vi "Lab Panel V5.10.vi"() -> ()   [LabVIEW 2013]
uses:
  <vilib>/Platform/TimedLoop/XDataNode/timing_clust.ctl
  <vilib>/Platform/TimedLoop/XDataNode/nitl_modes.ctl
  <vilib>/Platform/TimedLoop/XDataNode/wakeup.ctl
  Global display 4.vi
  Global display 3.vi
  Global display 1.vi
  Global 1.vi
  Global display 2.vi
  <vilib>/platform/TimedLoop/XDataNode/XDataNode.xnode
  <vilib>/Platform/TimedLoop/XDataNode/XDNodeRunTimeDep.lvlib
panel:
  out "Simulate IND":bool
  out "Amb Tp":dbl format="%#.0f"
  out "Tp Ut":dbl
  out "network error":bool
  out "TEMP":bool
  out "AI":bool
  in  "stop all":bool
  in  "ADMIN":bool
  in  "Tab Control 2":T1(tab)
  out "SIG LAB05-2":T2 {"PF" format="%.2f"; "AMPS" format="%.1f"}
  out "SIG LAB05-1":T2 {"PF" format="%.2f"; "AMPS" format="%.1f"}
  out "SIG LAB04-2":T2 {"PF" format="%.2f"; "AMPS" format="%.1f"}
  out "SIG LAB04-1":T2 {"PF" format="%.2f"; "AMPS" format="%.1f"}
  out "SIG LAB03-2":T2 {"PF" format="%.2f"; "AMPS" format="%.1f"}
  out "SIG LAB03-1":T2 {"PF" format="%.2f"; "AMPS" format="%.1f"}
  out "SIG LAB02-2":T2 {"PF" format="%.2f"; "AMPS" format="%.1f"}
  in  "RUN LAB01-1":bool
  in  "O/I  LAB05-1":bool
  in  "O/I  LAB05-2":bool
  in  "O/I  LAB04-1":bool
  in  "O/I  LAB04-2":bool
  in  "O/I  LAB02-1":bool
  in  "O/I  LAB02-2":bool
  in  "O/I  LAB01-2":bool
  in  "O/I  LAB01-1":bool
  in  "O/I  LAB03-1":bool
  in  "RUN LAB05-2":bool
  in  "RUN LAB05-1":bool
  in  "RUN LAB04-2":bool
  in  "RUN LAB04-1":bool
  in  "RUN LAB03-2":bool
  in  "RUN LAB03-1":bool
  in  "RUN LAB02-2":bool
  in  "RUN LAB02-1":bool
  in  "RUN LAB01-2":bool
  in  "SELECT LAB05-2":T3(radio)
  in  "SELECT LAB05-1":T3(radio)
  in  "SELECT LAB04-2":T3(radio)
  in  "SELECT LAB04-1":T3(radio)
  in  "SELECT LAB03-2":T3(radio)
  in  "SELECT LAB03-1":T3(radio)
  in  "SELECT LAB02-2":T3(radio)
  in  "SELECT LAB02-1":T3(radio)
  in  "SELECT LAB01-2":T3(radio)
  in  "SELECT LAB01-1":T3(radio)
  in  "O/I  LAB03-2":bool
  out "SIG LAB01-1":T2 {"PF" format="%.2f"; "AMPS" format="%.1f"}
  out "SIG LAB01-2":T2 {"PF" format="%.2f"; "AMPS" format="%.1f"}
  out "SIG LAB02-1":T2 {"PF" format="%.2f"; "AMPS" format="%.1f"}
  out "DISP LAB05-2":T4 {"MINS" format="%.2g"}
  out "DISP LAB05-1":T4 {"MINS" format="%.2g"}
  out "DISP LAB04-2":T4 {"MINS" format="%.2g"}
  out "DISP LAB04-1":T4 {"MINS" format="%.2g"}
  out "DISP LAB03-2":T4 {"MINS" format="%.2g"}
  out "DISP LAB03-1":T4 {"MINS" format="%.2g"}
  in  "SET LAB05-2":T5={"NAME"="", "DESCRIPTION"="", "CYCLES"=5.0, "T-RISE mins"=0.0, "T-RISE deg C"=0.0} {"CYCLES" min=5.0 step=1.0}
  in  "SET LAB05-1":T5={"NAME"="", "DESCRIPTION"="", "CYCLES"=5.0, "T-RISE mins"=0.0, "T-RISE deg C"=0.0} {"CYCLES" min=5.0 step=1.0}
  in  "SET LAB04-2":T5={"NAME"="", "DESCRIPTION"="", "CYCLES"=5.0, "T-RISE mins"=0.0, "T-RISE deg C"=0.0} {"CYCLES" min=5.0 step=1.0}
  in  "SET LAB04-1":T5={"NAME"="", "DESCRIPTION"="", "CYCLES"=5.0, "T-RISE mins"=0.0, "T-RISE deg C"=0.0} {"CYCLES" min=5.0 step=1.0}
  in  "SET LAB03-2":T5={"NAME"="", "DESCRIPTION"="", "CYCLES"=5.0, "T-RISE mins"=0.0, "T-RISE deg C"=0.0} {"CYCLES" min=5.0 step=1.0}
  in  "SET LAB03-1":T5={"NAME"="", "DESCRIPTION"="", "CYCLES"=5.0, "T-RISE mins"=0.0, "T-RISE deg C"=0.0} {"CYCLES" min=5.0 step=1.0}
  out "DISP LAB02-2":T4 {"MINS" format="%.2g"}
  out "DISP LAB02-1":T4 {"MINS" format="%.2g"}
  in  "SET LAB02-2":T5={"NAME"="", "DESCRIPTION"="", "CYCLES"=5.0, "T-RISE mins"=0.0, "T-RISE deg C"=0.0} {"CYCLES" min=5.0 step=1.0}
  in  "SET LAB02-1":T5={"NAME"="", "DESCRIPTION"="", "CYCLES"=5.0, "T-RISE mins"=0.0, "T-RISE deg C"=0.0} {"CYCLES" min=5.0 step=1.0}
  out "RESULT LAB05-2":bool
  out "RESULT LAB05-1":bool
  out "RESULT LAB04-2":bool
  out "RESULT LAB04-1":bool
  out "RESULT LAB03-2":bool
  out "RESULT LAB03-1":bool
  out "RESULT LAB02-2":bool
  out "RESULT LAB02-1":bool
  out "RESULT LAB01-2":bool
  out "RESULT LAB01-1":bool
  in  "SET LAB01-1":T5={"NAME"="", "DESCRIPTION"="", "CYCLES"=5.0, "T-RISE mins"=0.0, "T-RISE deg C"=0.0} {"CYCLES" min=5.0 step=1.0}
  in  "SET LAB01-2":T5={"NAME"="", "DESCRIPTION"="", "CYCLES"=5.0, "T-RISE mins"=0.0, "T-RISE deg C"=0.0} {"CYCLES" min=5.0 step=1.0}
  out "DISP LAB01-1":T4 {"MINS" format="%.2g"}
  out "DISP LAB01-2":T4 {"MINS" format="%.2f"}
  out "TEMP RISE LAB05-2":cluster{"TL":dbl, "TN":dbl}
  out "TEMP RISE LAB05-1":cluster{"TL":dbl, "TN":dbl}
  out "TEMP RISE LAB04-2":cluster{"TL":dbl, "TN":dbl}
  out "TEMP RISE LAB04-1":cluster{"TL":dbl, "TN":dbl}
  out "TEMP RISE LAB03-2":cluster{"TL":dbl, "TN":dbl}
  out "TEMP RISE LAB03-1":cluster{"TL":dbl, "TN":dbl}
  out "TEMP RISE LAB02-2":cluster{"TL":dbl, "TN":dbl}
  out "TEMP RISE LAB02-1":cluster{"TL":dbl, "TN":dbl}
  out "TEMP RISE LAB01-2":cluster{"TL":dbl, "TN":dbl}
  out "TEMP RISE LAB01-1":cluster{"TL":dbl, "TN":dbl}
  out "JIG LAB05-2":bool
  out "JIG LAB05-1":bool
  out "JIG LAB04-2":bool
  out "JIG LAB04-1":bool
  out "JIG LAB03-2":bool
  out "JIG LAB03-1":bool
  out "JIG LAB02-2":bool
  out "JIG LAB02-1":bool
  out "JIG LAB01-2":bool
  out "JIG LAB01-1":bool
  out "TEMP START LAB01-1":cluster{"TL":dbl, "TN":dbl}
  out "TEMP START LAB02-1":cluster{"TL":dbl, "TN":dbl}
  out "TEMP START LAB03-1":cluster{"TL":dbl, "TN":dbl}
  out "TEMP START LAB04-1":cluster{"TL":dbl, "TN":dbl}
  out "TEMP START LAB01-2":cluster{"TL":dbl, "TN":dbl}
  out "TEMP START LAB02-2":cluster{"TL":dbl, "TN":dbl}
  out "TEMP START LAB03-2":cluster{"TL":dbl, "TN":dbl}
  out "TEMP START LAB04-2":cluster{"TL":dbl, "TN":dbl}
  out "TEMP START LAB05-2":cluster{"TL":dbl, "TN":dbl}
  out "TEMP START LAB05-1":cluster{"TL":dbl, "TN":dbl}
  out "LOG LAB05-2":string
  out "LOG LAB04-2":string
  out "LOG LAB03-2":string
  out "LOG LAB02-2":string
  out "LOG LAB01-2":string
  out "LOG LAB05-1":string
  out "LOG LAB04-1":string
  out "LOG LAB03-1":string
  out "LOG LAB02-1":string
  out "LOG LAB01-1":string
  in  "Tab charts":T6(tab)
  out "LAB01 VOLTS":dynamicdata(graph)
  out "LAB01 AMPS":dynamicdata(graph)
  out "LAB01 deg C":dynamicdata(graph)
  out "LAB02 VOLTS":dynamicdata(graph)
  out "LAB02 AMPS":dynamicdata(graph)
  out "LAB02 deg C":dynamicdata(graph)
  out "LAB03 VOLTS":dynamicdata(graph)
  out "LAB03 AMPS":dynamicdata(graph)
  out "LAB03 deg C":dynamicdata(graph)
  out "LAB04 VOLTS":dynamicdata(graph)
  out "LAB04 AMPS":dynamicdata(graph)
  out "LAB04 deg C":dynamicdata(graph)
  out "LAB05 VOLTS":dynamicdata(graph)
  out "LAB05 AMPS":dynamicdata(graph)
  out "LAB05 deg C":dynamicdata(graph)
  out "Resets Done":dbl
  out "Error USB #2":bool
  out "Error USB #1":bool
  out "Error USB #0":bool
  in  "MAIL SETTINGS":T7
  out "MAIL REPORT":string
  in  "TO (string):":string
  in  "Send Mail Now":bool
  in  "Auto Mail Send":bool
  in  "Network Directory":path
  in  "JIG ON TIME (S)":dbl=1.0 min=1.0 max=10.0 step=0.5 format="%.1g"
  in  "JIG OFF TIME (S)":dbl=2.0 min=2.0 max=10.0 step=0.5 format="%.1g"
  in  "Reset Measuring":bool
  out "JIG RELAY CYCLES":T8
  out "ON L05-2":cluster{"amps":dbl, "volts":dbl, "pf":dbl}
  out "ON L05-1":cluster{"amps":dbl, "volts":dbl, "pf":dbl}
  out "FAIL LAB05-2":cluster{"LO":dbl, "HI":dbl}
  out "FAIL LAB05-1":cluster{"LO":dbl, "HI":dbl}
  out "FAIL LAB04-2":cluster{"LO":dbl, "HI":dbl}
  out "FAIL LAB04-1":cluster{"LO":dbl, "HI":dbl}
  out "FAIL LAB03-2":cluster{"LO":dbl, "HI":dbl}
  out "FAIL LAB03-1":cluster{"LO":dbl, "HI":dbl}
  out "FAIL LAB02-2":cluster{"LO":dbl, "HI":dbl}
  out "FAIL LAB02-1":cluster{"LO":dbl, "HI":dbl}
  out "FAIL LAB01-2":cluster{"LO":dbl, "HI":dbl}
  out "FAIL LAB01-1":cluster{"LO":dbl, "HI":dbl}
  out "ON L01-1":cluster{"amps":dbl, "volts":dbl, "pf":dbl}
  out "ON L01-2":cluster{"amps":dbl, "volts":dbl, "pf":dbl}
  out "ON L02-1":cluster{"amps":dbl, "volts":dbl, "pf":dbl}
  out "ON L02-2":cluster{"amps":dbl, "volts":dbl, "pf":dbl}
  out "ON L03-1":cluster{"amps":dbl, "volts":dbl, "pf":dbl}
  out "ON L03-2":cluster{"amps":dbl, "volts":dbl, "pf":dbl}
  out "ON L04-1":cluster{"amps":dbl, "volts":dbl, "pf":dbl}
  out "ON L04-2":cluster{"amps":dbl, "volts":dbl, "pf":dbl}
  out "TEMP LA05":T9
  out "TEMP LA04":T9
  out "TEMP LA03":T9
  out "TEMP LA02":T9
  out "TEMP LA01":T9
  out "Ref deg C":dbl format="%#.0f"
  out "Panel #":dbl
  in  "Mail Test File To:":string
  in  "Mail Test Fail":bool
  out "graph flag":bool
  in  "Temp Test Cal":dbl
  in  "Amps Fail level":dbl
  in  "Fail Loops":dbl
  out "Save JC":bool
  out "simulate":bool
  in  "Temp Value":dbl
  in  "Temp Delay Lps":dbl
  in  "SAMPLES":dbl
  in  "RATE (Hz)":dbl
  in  "JIG TEST":T10
  in  "C drive data root dir":path
  out "run lab05-2":bool
  out "run lab05-1":bool
  out "run lab04-2":bool
  out "run lab04-1":bool
  out "run lab03-2":bool
  out "run lab03-1":bool
  out "run lab02-2":bool
  out "run lab02-1":bool
  out "run lab01-2":bool
  out "run lab01-1":bool
  in  "Tab Control":T11(tab)
  out "LAB01-2 (GRAPH)":dynamicdata(graph)
  out "LAB01-1 (GRAPH)":dynamicdata(graph)
  out "LAB02-2 (GRAPH)":dynamicdata(graph)
  out "LAB02-1 (GRAPH)":dynamicdata(graph)
  out "LAB03-2 (GRAPH)":dynamicdata(graph)
  out "LAB03-1 (GRAPH)":dynamicdata(graph)
  out "LAB04-2 (GRAPH)":dynamicdata(graph)
  out "LAB04-1 (GRAPH)":dynamicdata(graph)
  out "LAB05-2 (GRAPH)":dynamicdata(graph)
  out "LAB05-1 (GRAPH)":dynamicdata(graph)
  out "LAB05 TEMP":T12
  out "LAB04 TEMP":T12
  out "LAB02 TEMP":T12
  out "LAB01 TEMP":T12
  out "LAB03 TEMP":T12
  out "Analog error":bool
  in  "Ambient Volts":dbl format="%.2f"
  in  "PF":dbl min=0.0 max=1.0 step=0.1 format="%#.1f"
  in  "VOLTS":dbl
  in  "OFF amps":dbl min=0.0 max=100.0 step=0.1 format="%#.1f"
  in  "ON amps":dbl
  in  "LAB deg C":T13
  out "AI loop time":dbl format="%.6g"
  out "loops":dbl
  in  "loop  delay(mS)":dbl
  out "on loops":dbl
  out "off loops":dbl
  out "jig cycle":dbl
  out "TDMS LAB01-1":refnum<k34>
  out "data file error":errorcluster
  out "TDMS LAB02-1":refnum<k34>
  out "TDMS LAB01-2":refnum<k34>
  out "TDMS LAB02-2":refnum<k34>
  out "TDMS LAB03-1":refnum<k34>
  out "TDMS LAB03-2":refnum<k34>
  out "TDMS LAB04-1":refnum<k34>
  out "TDMS LAB04-2":refnum<k34>
  out "TDMS LAB05-1":refnum<k34>
  out "TDMS LAB05-2":refnum<k34>
  out "mail control":string
  out "File Time Stamp":timestamp
  in  "stop":bool
  in  "Select COM port":refnum<visa-resource-name>="COM6"
  out "COM port":refnum<visa-resource-name>="COM6"
  out "deg C (volts)":dbl
  out "TEMP REF cal":dbl
  out "CAL LAB01":T14 {"2 (TN) cal" min=0.0 step=0.01 format="%.2f"; "2 (TL) cal" min=0.0 step=0.01 format="%.2f"; "2 (PF) cal" min=0.0 step=0.01 format="%.2f"; "2 (V) cal" min=0.0 step=0.01 format="%.2f"; "2 (A) cal" min=0.0 step=0.01 format="%.2f"; "1 (TN) cal" min=0.0 step=0.01 format="%.2f"; "1 (TL) cal" min=0.0 step=0.01 format="%.2f"; "1 (PF) cal" min=0.0 step=0.01 format="%.2f"; "1 (V) cal" min=0.0 step=0.01 format="%.2f"; "1  (A) cal" min=0.0 step=0.01 format="%.2f"}
  out "CAL LAB03":T14 {"2 (TN) cal" min=0.0 step=0.01 format="%.2f"; "2 (TL) cal" min=0.0 step=0.01 format="%.2f"; "2 (PF) cal" min=0.0 step=0.01 format="%.2f"; "2 (V) cal" min=0.0 step=0.01 format="%.2f"; "2 (A) cal" min=0.0 step=0.01 format="%.2f"; "1 (TN) cal" min=0.0 step=0.01 format="%.2f"; "1 (TL) cal" min=0.0 step=0.01 format="%.2f"; "1 (PF) cal" min=0.0 step=0.01 format="%.2f"; "1 (V) cal" min=0.0 step=0.01 format="%.2f"; "1  (A) cal" min=0.0 step=0.01 format="%.2f"}
  out "CAL LAB02":T15 {"2 (TN) cal" min=0.0 step=0.01 format="%.2f"; "2 (TL) cal" min=0.0 step=0.01 format="%.2f"; "2 (PF) cal" min=0.0 step=0.01 format="%.2f"; "2 (V) cal" min=0.0 step=0.01 format="%.2f"; "2 (A) cal" min=0.0 step=0.01 format="%.2f"; "1 (TN) cal" min=0.0 step=0.01 format="%.2f"; "1 (TL) cal" min=0.0 step=0.01 format="%.2f"; "1 (PF) cal" min=0.0 step=0.01 format="%.2f"; "1 (V) cal" min=0.0 step=0.01 format="%.2f"; "1 (A) cal" min=0.0 step=0.01 format="%.2f"}
  out "CAL LAB05":T14 {"2 (TN) cal" min=0.0 step=0.01 format="%.2f"; "2 (TL) cal" min=0.0 step=0.01 format="%.2f"; "2 (PF) cal" min=0.0 step=0.01 format="%.2f"; "2 (V) cal" min=0.0 step=0.01 format="%.2f"; "2 (A) cal" min=0.0 step=0.01 format="%.2f"; "1 (TN) cal" min=0.0 step=0.01 format="%.2f"; "1 (TL) cal" min=0.0 step=0.01 format="%.2f"; "1 (PF) cal" min=0.0 step=0.01 format="%.2f"; "1 (V) cal" min=0.0 step=0.01 format="%.2f"; "1  (A) cal" min=0.0 step=0.01 format="%.2f"}
  out "CAL LAB04":T14 {"2 (TN) cal" min=0.0 step=0.01 format="%.2f"; "2 (TL) cal" min=0.0 step=0.01 format="%.2f"; "2 (PF) cal" min=0.0 step=0.01 format="%.2f"; "2 (V) cal" min=0.0 step=0.01 format="%.2f"; "2 (A) cal" min=0.0 step=0.01 format="%.2f"; "1 (TN) cal" min=0.0 step=0.01 format="%.2f"; "1 (TL) cal" min=0.0 step=0.01 format="%.2f"; "1 (PF) cal" min=0.0 step=0.01 format="%.2f"; "1 (V) cal" min=0.0 step=0.01 format="%.2f"; "1  (A) cal" min=0.0 step=0.01 format="%.2f"}
  out "cal file error out":errorcluster
  in  "SET (cal)":bool
  # "LAB01"
  # "LAB02"
  # "LAB03"
  # "LAB04"
  # "LAB05"
  # "LAB01"
  # "LAB02"
  # "LAB03"
  # "LAB04"
  # "LAB05"
  # "PANEL ID / DATE / TIME / NAME / DESCRIPTION / CYCLES / TEST TIME / STATUS"
  # "PANEL ID / DATE / TIME / NAME / DESCRIPTION / CYCLES / TEST TIME / STATUS"
  # "(Enter recipients address seperated by comma)"
  # "JIG SET"
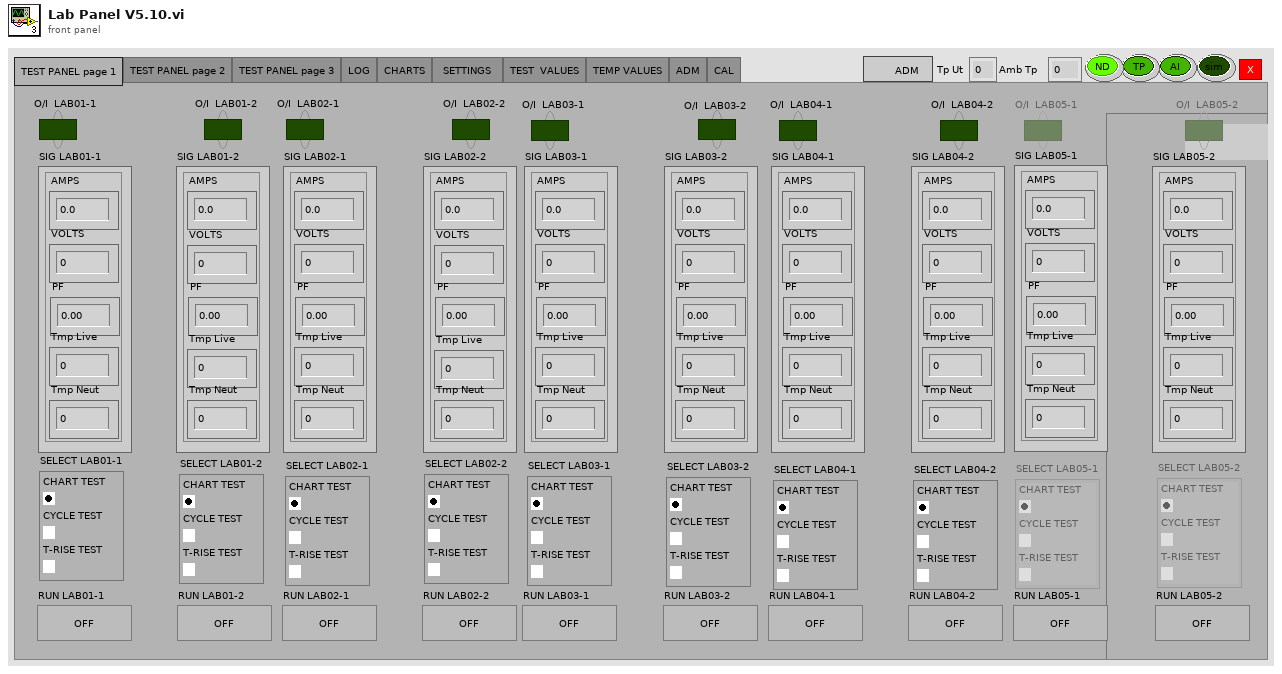
[diagram p1: front panel]
types:
  T1 = enum32{"TEST PANEL page 1", "TEST PANEL page 2", "TEST PANEL page 3", "LOG", "CHARTS", "SETTINGS   ", "TEST  VALUES", "TEMP VALUES", "ADM", "CAL"}
  T2 = cluster{"AMPS":dbl, "VOLTS":dbl, "PF":dbl, "Tmp Live":dbl, "Tmp Neut":dbl}
  T3 = enum32{"CHART TEST", "CYCLE TEST", "T-RISE TEST"}
  T4 = cluster{"CYCLE":dbl, "MINS":dbl, "STATUS":string}
  T5 = cluster{"NAME":string, "DESCRIPTION":string, "CYCLES":dbl, "T-RISE mins":dbl, "T-RISE deg C":dbl}
  T6 = enum32{"LAB01", "LAB02", "LAB03", "LAB04", "LAB05"}
  T7 = cluster{"OUT SERVER ADDRESS":string, "FROM ACCOUNT":string, "USER NAME":string, "PASSWORD":string, "TEST MAIL":bool, "TEST MAIL STATUS":string, "mail error":errorcluster}
  T8 = cluster{"LAB01-1":dbl, "LAB01-2":dbl, "LAB02-1":dbl, "LAB02-2":dbl, "LAB03-1":dbl, "LAB03-2":dbl, "LAB04-1":dbl, "LAB04-2":dbl, "LAB05-1":dbl, "LAB05-2":dbl}
  T9 = cluster{"TL-1":dbl, "TN-1":dbl, "TL-2":dbl, "TN-2":dbl, "TL -1COUNT":dbl, "TN-1 COUNT":dbl, "TL-2 COUNT":dbl, "TN-2 COUNT":dbl}
  T10 = cluster{" LAB01-1":bool, " LAB01-2":bool, "LAB02-1":bool, " LAB02-2":bool, "LAB03-1":bool, "LAB03-2":bool, "LAB04-1":bool, "LAB04-2":bool, "LAB05-1":bool, "LAB05-2":bool}
  T11 = enum32{"LAB01", "LAB02", "LAB03", "LAB04", "LAB05", "TEMPERATURE", "ERROR", "Simulate"}
  T12 = cluster{"T1 Live":dbl, "T1 Neut":dbl, "T2 Live":dbl, "T2 Neut":dbl, "ID":dbl, "ER":dbl}
  T13 = cluster{"1 TL":dbl, "1 TN":dbl, "2 TL":dbl, "2 TN":dbl, "ID":dbl, "ER":dbl}
  T14 = cluster{"1  (A) cal":dbl, "1 (V) cal":dbl, "1 (PF) cal":dbl, "1 (TL) cal":dbl, "1 (TN) cal":dbl, "2 (A) cal":dbl, "2 (V) cal":dbl, "2 (PF) cal":dbl, "2 (TL) cal":dbl, "2 (TN) cal":dbl}
  T15 = cluster{"1 (A) cal":dbl, "1 (V) cal":dbl, "1 (PF) cal":dbl, "1 (TL) cal":dbl, "1 (TN) cal":dbl, "2 (A) cal":dbl, "2 (V) cal":dbl, "2 (PF) cal":dbl, "2 (TL) cal":dbl, "2 (TN) cal":dbl}
  T16 = enum8{"Enabled", "Disabled", "Disabled and Grayed Out"}
  T17 = typedef "XDNodeRunTimeDep.lvlib/timing_clust.ctl" = cluster{"Expected End [f-1]":u64, "Actual End [f-1]":u64, "Finished Late? [f-1]":bool, "Expected End [i-1]":u64, "Actual End [i-1]":u64, "Finished Late? [i-1]":bool, "Expected Start [i]":u64, "Actual Start [i]":u64, "Expected Start [f]":u64, "Actual Start [f]":u64, "Source Name":string, "Structure Name":string, "Period":i64, "Deadline":i64, "Offset":i64, "Start":i64, "Priority":i32, "Timeout":i32, "Mode":T18, "Wakeup Reason":T19, "Error":errorcluster, "Source Type":string, "Secondary Source Type":string, "Global End Time":u64, "Global Start Time":u64, "Frame Duration":u64, "Iteration Duration":u64, "Assigned CPU":i32, "I/O Scan Engine Mode":u32}
  T18 = typedef "XDNodeRunTimeDep.lvlib/nitl_modes.ctl" = enum32{"No Change", "Process missed periods, maintain original phase", "Discard missed periods, maintain original phase", "Process missed periods, ignore original phase", "Discard missed periods, ignore original phase"}
  T19 = typedef "XDNodeRunTimeDep.lvlib/wakeup.ctl" = enum32{"Normal", "Aborted", "Asynchronous wakeup", "Timing source error", "Timed loop error", "Timeout"}
  T20 = enum16{"open", "open or create", "create or replace", "create", "open (read-only)"}
  T21 = enum16{"open", "replace", "create", "open or create", "replace or create", "replace or create with confirmation"}
  T22 = cluster{"SET LAB01-1":cluster{"NAME":string, "DESCRIPTION":string, "CYCLES":dbl, "T-RISE mins":dbl, "T-RISE deg C":dbl}, "SET LAB01-2":cluster{"NAME":string, "DESCRIPTION":string, "CYCLES":dbl, "T-RISE mins":dbl, "T-RISE deg C":dbl}, "SET LAB02-1":cluster{"NAME":string, "DESCRIPTION":string, "CYCLES":dbl, "T-RISE mins":dbl, "T-RISE deg C":dbl}, "SET LAB02-2":cluster{"NAME":string, "DESCRIPTION":string, "CYCLES":dbl, "T-RISE mins":dbl, "T-RISE deg C":dbl}, "SET LAB03-1":cluster{"NAME":string, "DESCRIPTION":string, "CYCLES":dbl, "T-RISE mins":dbl, "T-RISE deg C":dbl}, "SET LAB03-2":cluster{"NAME":string, "DESCRIPTION":string, "CYCLES":dbl, "T-RISE mins":dbl, "T-RISE deg C":dbl}, "SET LAB04-1":cluster{"NAME":string, "DESCRIPTION":string, "CYCLES":dbl, "T-RISE mins":dbl, "T-RISE deg C":dbl}, "SET LAB04-2":cluster{"NAME":string, "DESCRIPTION":string, "CYCLES":dbl, "T-RISE mins":dbl, "T-RISE deg C":dbl}, "SET LAB05-1":cluster{"NAME":string, "DESCRIPTION":string, "CYCLES":dbl, "T-RISE mins":dbl, "T-RISE deg C":dbl}, "SET LAB05-2":cluster{"NAME":string, "DESCRIPTION":string, "CYCLES":dbl, "T-RISE mins":dbl, "T-RISE deg C":dbl}, "Network Directory":path, "C drive data root dir":path, "RATE (Hz)":dbl, "SAMPLES":dbl, "Select COM port":refnum<visa-resource-name>, "Temp Delay Lps":dbl, "Temp Value":dbl, "Fail Loops":dbl, "Temp Test Cal":dbl, "Amps Fail level":dbl, "Mail Test File To:":string, "Mail Test Fail":bool}
  T23 = cluster{"MAIL SETTINGS":cluster{"OUT SERVER ADDRESS":string, "FROM ACCOUNT":string, "USER NAME":string, "PASSWORD":string, "TEST MAIL":bool, "TEST MAIL STATUS":string, "mail error":errorcluster}, "Auto Mail Send":bool, string}
  T24 = cluster{"T1":dbl, "T2":dbl, "T3":dbl, "T4":dbl, "ID":dbl, "ER":dbl}
  T25 = cluster{"STATUS":string, "OUT SERVER ADDRESS":string, "FROM ACCOUNT":string, "Mail Test File To:":string, "Mail Test Fail":bool}
  T26 = cluster{"LAB01-1 (A)":dbl, "LAB01-1 (V)":dbl, "LAB01-1 (PF)":dbl, "LAB01-2 (A)":dbl, "LAB01-2 (V)":dbl, "LAB01-2 (PF)":dbl}
  T27 = cluster{"LAB02-1 (A)":dbl, "LAB02-1 (V)":dbl, "LAB02-1 (PF)":dbl, "LAB02-2 (A)":dbl, "LAB02-2 (V)":dbl, "LAB02-2 (PF)":dbl}
  T28 = cluster{"LAB03-1 (A)":dbl, "LAB03-1 (V)":dbl, "LAB03-1 (PF)":dbl, "LAB03-2 (A)":dbl, "LAB03-2 (V)":dbl, "LAB03-2 (PF)":dbl}
  T29 = cluster{"LAB04-1 (A)":dbl, "LAB04-1 (V)":dbl, "LAB04-1 (PF)":dbl, "LAB04-2 (A)":dbl, "LAB04-2 (V)":dbl, "LAB04-2 (PF)":dbl}
  T30 = cluster{"LAB05-1 (A)":dbl, "LAB05-1 (V)":dbl, "LAB05-1 (PF)":dbl, "LAB05-2 (A)":dbl, "LAB05-2 (V)":dbl, "LAB05-2 (PF)":dbl}
  T31 = cluster{"OFF amps":dbl, "VOLTS":dbl, "PF":dbl, "OFF amps":dbl, "VOLTS":dbl, "PF":dbl}
  T32 = cluster{"FAIL LAB01-1":cluster{"LO":dbl, "HI":dbl}, "SIG LAB01-1":cluster{"AMPS":dbl, "VOLTS":dbl, "PF":dbl, "Tmp Live":dbl, "Tmp Neut":dbl}, "TEMP START LAB01-1":cluster{"TL":dbl, "TN":dbl}, "DISP LAB01-1":cluster{"CYCLE":dbl, "MINS":dbl, "STATUS":string}, "SET LAB01-1":cluster{"NAME":string, "DESCRIPTION":string, "CYCLES":dbl, "T-RISE mins":dbl, "T-RISE deg C":dbl}, "TDMS LAB01-1":refnum<k34>}
  T33 = cluster{"FAIL LAB01-2":cluster{"LO":dbl, "HI":dbl}, "SIG LAB01-2":cluster{"AMPS":dbl, "VOLTS":dbl, "PF":dbl, "Tmp Live":dbl, "Tmp Neut":dbl}, "TEMP START LAB01-2":cluster{"TL":dbl, "TN":dbl}, "DISP LAB01-2":cluster{"CYCLE":dbl, "MINS":dbl, "STATUS":string}, "SET LAB01-2":cluster{"NAME":string, "DESCRIPTION":string, "CYCLES":dbl, "T-RISE mins":dbl, "T-RISE deg C":dbl}, "TDMS LAB01-2":refnum<k34>}
  T34 = cluster{"FAIL LAB02-1":cluster{"LO":dbl, "HI":dbl}, "SIG LAB02-1":cluster{"AMPS":dbl, "VOLTS":dbl, "PF":dbl, "Tmp Live":dbl, "Tmp Neut":dbl}, "TEMP START LAB02-1":cluster{"TL":dbl, "TN":dbl}, "DISP LAB02-1":cluster{"CYCLE":dbl, "MINS":dbl, "STATUS":string}, "SET LAB02-1":cluster{"NAME":string, "DESCRIPTION":string, "CYCLES":dbl, "T-RISE mins":dbl, "T-RISE deg C":dbl}, "TDMS LAB02-1":refnum<k34>}
  T35 = cluster{"FAIL LAB02-2":cluster{"LO":dbl, "HI":dbl}, "SIG LAB02-2":cluster{"AMPS":dbl, "VOLTS":dbl, "PF":dbl, "Tmp Live":dbl, "Tmp Neut":dbl}, "TEMP START LAB02-2":cluster{"TL":dbl, "TN":dbl}, "DISP LAB02-2":cluster{"CYCLE":dbl, "MINS":dbl, "STATUS":string}, "SET LAB02-2":cluster{"NAME":string, "DESCRIPTION":string, "CYCLES":dbl, "T-RISE mins":dbl, "T-RISE deg C":dbl}, "TDMS LAB02-2":refnum<k34>}
  T36 = cluster{"FAIL LAB03-1":cluster{"LO":dbl, "HI":dbl}, "SIG LAB03-1":cluster{"AMPS":dbl, "VOLTS":dbl, "PF":dbl, "Tmp Live":dbl, "Tmp Neut":dbl}, "TEMP START LAB03-1":cluster{"TL":dbl, "TN":dbl}, "DISP LAB03-1":cluster{"CYCLE":dbl, "MINS":dbl, "STATUS":string}, "SET LAB03-1":cluster{"NAME":string, "DESCRIPTION":string, "CYCLES":dbl, "T-RISE mins":dbl, "T-RISE deg C":dbl}, "TDMS LAB03-1":refnum<k34>}
  T37 = cluster{"FAIL LAB03-2":cluster{"LO":dbl, "HI":dbl}, "SIG LAB03-2":cluster{"AMPS":dbl, "VOLTS":dbl, "PF":dbl, "Tmp Live":dbl, "Tmp Neut":dbl}, "TEMP START LAB03-2":cluster{"TL":dbl, "TN":dbl}, "DISP LAB03-2":cluster{"CYCLE":dbl, "MINS":dbl, "STATUS":string}, "SET LAB03-2":cluster{"NAME":string, "DESCRIPTION":string, "CYCLES":dbl, "T-RISE mins":dbl, "T-RISE deg C":dbl}, "TDMS LAB03-2":refnum<k34>}
  T38 = cluster{"FAIL LAB04-1":cluster{"LO":dbl, "HI":dbl}, "SIG LAB04-1":cluster{"AMPS":dbl, "VOLTS":dbl, "PF":dbl, "Tmp Live":dbl, "Tmp Neut":dbl}, "TEMP START LAB04-1":cluster{"TL":dbl, "TN":dbl}, "DISP LAB04-1":cluster{"CYCLE":dbl, "MINS":dbl, "STATUS":string}, "SET LAB04-1":cluster{"NAME":string, "DESCRIPTION":string, "CYCLES":dbl, "T-RISE mins":dbl, "T-RISE deg C":dbl}, "TDMS LAB04-1":refnum<k34>}
  T39 = cluster{"FAIL LAB04-2":cluster{"LO":dbl, "HI":dbl}, "SIG LAB04-2":cluster{"AMPS":dbl, "VOLTS":dbl, "PF":dbl, "Tmp Live":dbl, "Tmp Neut":dbl}, "TEMP START LAB04-2":cluster{"TL":dbl, "TN":dbl}, "DISP LAB04-2":cluster{"CYCLE":dbl, "MINS":dbl, "STATUS":string}, "SET LAB04-2":cluster{"NAME":string, "DESCRIPTION":string, "CYCLES":dbl, "T-RISE mins":dbl, "T-RISE deg C":dbl}, "TDMS LAB04-2":refnum<k34>}
  T40 = cluster{"FAIL LAB05-1":cluster{"LO":dbl, "HI":dbl}, "SIG LAB05-1":cluster{"AMPS":dbl, "VOLTS":dbl, "PF":dbl, "Tmp Live":dbl, "Tmp Neut":dbl}, "TEMP START LAB05-1":cluster{"TL":dbl, "TN":dbl}, "DISP LAB05-1":cluster{"CYCLE":dbl, "MINS":dbl, "STATUS":string}, "SET LAB05-1":cluster{"NAME":string, "DESCRIPTION":string, "CYCLES":dbl, "T-RISE mins":dbl, "T-RISE deg C":dbl}, "TDMS LAB05-1":refnum<k34>}
  T41 = cluster{"FAIL LAB05-2":cluster{"LO":dbl, "HI":dbl}, "SIG LAB05-2":cluster{"AMPS":dbl, "VOLTS":dbl, "PF":dbl, "Tmp Live":dbl, "Tmp Neut":dbl}, "TEMP START LAB05-2":cluster{"TL":dbl, "TN":dbl}, "DISP LAB05-2":cluster{"CYCLE":dbl, "MINS":dbl, "STATUS":string}, "SET LAB05-2":cluster{"NAME":string, "DESCRIPTION":string, "CYCLES":dbl, "T-RISE mins":dbl, "T-RISE deg C":dbl}, "TDMS LAB05-2":refnum<k34>}
  T42 = cluster{"MAIL SETTINGS":cluster{"OUT SERVER ADDRESS":string, "FROM ACCOUNT":string, "USER NAME":string, "PASSWORD":string, "TEST MAIL":bool, "TEST MAIL STATUS":string, "mail error":errorcluster}, "Auto Mail Send":bool, "TO (string):":string}
  T43 = cluster{"TP1-L":dbl, "TP1-N":dbl, "TP2-L":dbl, "TP2-N":dbl, "TP1-L COUNT":dbl, "TP1-N COUNT":dbl, "TP2-L COUNT":dbl, "TP2-N COUNT":dbl}
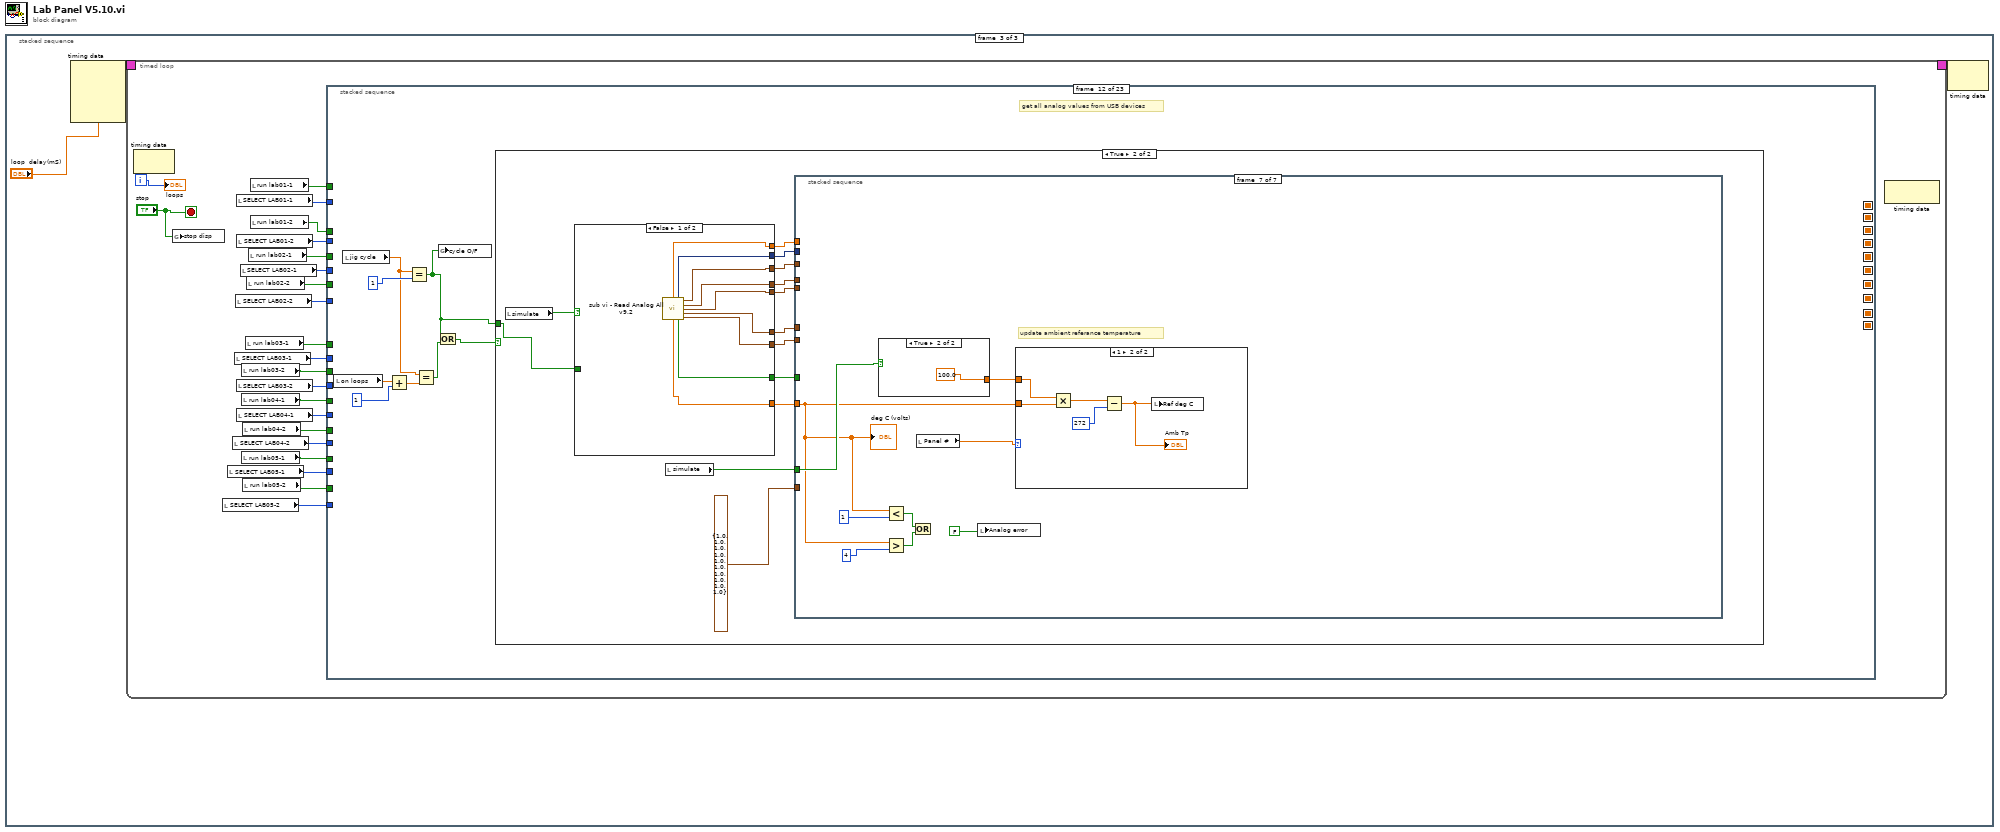
[diagram p0: block diagram]
diagram:
  n1 = stacked-sequence {
    frame #0 {
      n2 = local write "loop  delay(mS)"(500) -> ()
      n3 = local write "Save JC"(FALSE) -> ()
      "jig cycle" <- 0
    }
    frame #1 {
      # "do 1st time set up"
      n4 = stacked-sequence {
        frame #0 {
          # "disable front panel while 1st time set up is being done"
          n5 = disable-structure shown="Enabled" {
            frame Enabled {
              n6 = property on="Tab Control 2" class="TabCtl (strict)"() -> ("Pages"=w10:refnum<vi>[])  [unwired: 2 in, 2 out]
              n7 = Index Array(array=w10, index=8) -> (element=w8:refnum<vi>)
              n8 = property class="Page"(reference=w8, "PageVis"=FALSE) -> ()  [unwired: 1 in, 2 out]
            }
            frame Disabled {
            }
          }
          n9 = property on="Tab Control 2" class="TabCtl (strict)"("Value"=0) -> ()  [unwired: 2 in, 2 out]
          n10 = local write "ADMIN"(FALSE) -> ()
          n11 = property on="Tab Control 2" class="TabCtl (strict)"("DisabledEnum"=T16."Disabled and Grayed Out" ("Disabled")) -> ()  [unwired: 2 in, 2 out]
        }
        frame #1 {
          # "get calibration values"
          n12 = call "sub vi - get calibration values v1.vi"() -> ("TEMP REF CAL"=w11:dbl, "LAB01 (CAL)"=→"CAL LAB01":T14, "LAB02 (CAL)"=→"CAL LAB02":T15, "LAB03 (CAL)"=→"CAL LAB03":T14, "LAB04 (CAL)"=→"CAL LAB04":T14, "calibration file error out"=→"cal file error out":errorcluster, "LAB05 (CAL)"=→"CAL LAB05":T14)  [unwired: 9 in]
          n13 = local write "TEMP REF cal"(w11) -> ()
        }
        frame #2 {
          # "get last saved test settings from file"
          n14 = local read "Network Directory"() -> (w40:path)
          n15 = local read "C drive data root dir"() -> (w38:path)
          n16 = local read "SET LAB05-2"() -> (w70:T5)
          n17 = local read "SET LAB05-1"() -> (w71:T5)
          n18 = local read "SAMPLES"() -> (w36:dbl)
          n19 = local read "SET LAB04-2"() -> (w72:T5)
          n20 = local read "RATE (Hz)"() -> (w37:dbl)
          n21 = local read "SET LAB03-2"() -> (w69:T5)
          n22 = local read "SET LAB04-1"() -> (w73:T5)
          n23 = local read "SET LAB03-1"() -> (w68:T5)
          n24 = local read "SET LAB02-2"() -> (w67:T5)
          n25 = local read "SET LAB02-1"() -> (w66:T5)
          n26 = local read "SET LAB01-2"() -> (w65:T5)
          n27 = local read "SET LAB01-1"() -> (w64:T5)
          n28 = local read "Select COM port"() -> (w32:refnum<visa-resource-name>)
          n29 = local read "Temp Delay Lps"() -> (w31:dbl)
          n30 = local read "Mail Test File To:"() -> (w21:string)
          n31 = local read "Temp Value"() -> (w30:dbl)
          n32 = local read "Temp Test Cal"() -> (w25:dbl)
          n33 = local read "Amps Fail level"() -> (w24:dbl)
          n34 = local read "Fail Loops"() -> (w27:dbl)
          n35 = local read "Mail Test Fail"() -> (w19:bool)
          n36 = Bundle("SET LAB01-1"=w64, "SET LAB01-2"=w65, "SET LAB02-1"=w66, "SET LAB02-2"=w67, "SET LAB03-1"=w68, "SET LAB03-2"=w69, "SET LAB04-1"=w73, "SET LAB04-2"=w72, "SET LAB05-1"=w71, "SET LAB05-2"=w70, "Network Directory"=w40, "C drive data root dir"=w38, "RATE (Hz)"=w37, "SAMPLES"=w36, "Select COM port"=w32, "Temp Delay Lps"=w31, "Temp Value"=w30, "Fail Loops"=w27, "Temp Test Cal"=w25, "Amps Fail level"=w24, "Mail Test File To:"=w21, "Mail Test Fail"=w19) -> (w57:T22)  [unwired: 1 in]
          n37 = String To Path(string="c:\\crabtree\\Set Up\\") -> (path=w61:path)
          n38 = Build Path(base path=w61, name or relative path="settings.bin") -> (appended path=w59:path)
          n39 = Create Folder(path (use dialog)=w61) -> (error out=w63:errorcluster)  [unwired: 2 in, 2 out]
          n40 = call <vilib>:"Clear Errors.vi"("error in (no error)"=w63) -> ()  [unwired: 6 in, 1 out]
          n41 = Open/Create/Replace File(file path (use dialog)=w59) -> (refnum out=w56:refnum<file>, error out=w58:errorcluster)  [unwired: 5 in, 1 out]
          n42 = Read from Binary File(5:w57, 8:w58, 11:w56) -> (0:w53:errorcluster, 2:w55:T22, 3:w54:refnum<file>)  [unwired: 3 in, 1 out]
          n43 = Unbundle(w55) -> ("SET LAB01-1"=w51:T5, "SET LAB01-2"=w50:T5, "SET LAB02-1"=w49:T5, "SET LAB02-2"=w48:T5, "SET LAB03-1"=w47:T5, "SET LAB03-2"=w46:T5, "SET LAB04-1"=w45:T5, "SET LAB04-2"=w44:T5, "SET LAB05-1"=w43:T5, "SET LAB05-2"=w42:T5, "Network Directory"=w41:path, "C drive data root dir"=w39:path, "RATE (Hz)"=w34:dbl, "SAMPLES"=w35:dbl, "Select COM port"=w33:refnum<visa-resource-name>, "Temp Delay Lps"=w29:dbl, "Temp Value"=w28:dbl, "Fail Loops"=w26:dbl, "Temp Test Cal"=w23:dbl, "Amps Fail level"=w22:dbl, "Mail Test File To:"=w20:string, "Mail Test Fail"=w18:bool)
          n44 = Close File(refnum=w54, error in=w53) -> (error out=w52:errorcluster)  [unwired: 1 out]
          n45 = local write "data file error"(w52) -> ()
          n46 = local write "Temp Test Cal"(w23) -> ()
          n47 = local write "Mail Test File To:"(w20) -> ()
          n48 = local write "Amps Fail level"(w22) -> ()
          n49 = local write "Mail Test Fail"(w18) -> ()
          n50 = local write "Fail Loops"(w26) -> ()
          n51 = local write "Temp Delay Lps"(w29) -> ()
          n52 = local write "C drive data root dir"(w39) -> ()
          n53 = local write "Temp Value"(w28) -> ()
          n54 = local write "Select COM port"(w33) -> ()
          n55 = local write "Network Directory"(w41) -> ()
          n56 = local write "SAMPLES"(w35) -> ()
          n57 = local write "RATE (Hz)"(w34) -> ()
          n58 = local write "SET LAB04-2"(w44) -> ()
          n59 = local write "SET LAB05-1"(w43) -> ()
          n60 = local write "SET LAB04-1"(w45) -> ()
          n61 = local write "SET LAB05-2"(w42) -> ()
          n62 = local write "SET LAB02-1"(w49) -> ()
          n63 = local write "SET LAB02-2"(w48) -> ()
          n64 = local write "SET LAB03-1"(w47) -> ()
          n65 = local write "SET LAB03-2"(w46) -> ()
          n66 = local write "SET LAB01-1"(w51) -> ()
          n67 = local write "SET LAB01-2"(w50) -> ()
        }
        frame #3 {
          # "get last saved jig cycles value from file"
          n68 = String To Path(string="c:\\crabtree\\Jig Cycles\\") -> (path=w83:path)
          n69 = Build Path(base path=w83, name or relative path="jigcycles.bin") -> (appended path=w81:path)
          n70 = Create Folder(path (use dialog)=w83) -> (error out=w85:errorcluster)  [unwired: 2 in, 2 out]
          n71 = call <vilib>:"Clear Errors.vi"("error in (no error)"=w85) -> ()  [unwired: 6 in, 1 out]
          n72 = Open/Create/Replace File(file path (use dialog)=w81) -> (refnum out=w79:refnum<file>, error out=w80:errorcluster)  [unwired: 5 in, 1 out]
          n73 = Read from Binary File(5:T8 {"LAB01-1"=0.0, "LAB01-2"=0.0, "LAB02-1"=0.0, "LAB02-2"=0.0, "LAB03-1"=0.0, "LAB03-2"=0.0, "LAB04-1"=0.0, "LAB04-2"=0.0, "LAB05-1"=0.0, "LAB05-2"=0.0} ("JIG RELAY CYCLES"), 8:w80, 11:w79) -> (0:w77:errorcluster, 2:w74:T8, 3:w78:refnum<file>)  [unwired: 3 in, 1 out]
          n74 = local write "JIG RELAY CYCLES"(w74) -> ()
          n75 = Close File(refnum=w78, error in=w77) -> (error out=w76:errorcluster)  [unwired: 1 out]
          n76 = local write "data file error"(w76) -> ()
        }
        frame #4 {
          # "get mail settings"
          n77 = local read "Auto Mail Send"() -> (w89:bool)
          n78 = local read "MAIL SETTINGS"() -> (w93:T7)
          n79 = String To Path(string="c:\\crabtree\\Set Up\\") -> (path=w101:path)
          n80 = Build Path(base path=w101, name or relative path="mail.bin") -> (appended path=w99:path)
          n81 = Create Folder(path (use dialog)=w101) -> (error out=w103:errorcluster)  [unwired: 2 in, 2 out]
          n82 = Bundle("MAIL SETTINGS"=w93, "Auto Mail Send"=w89, "") -> (w92:T23)  [unwired: 1 in]
          n83 = call <vilib>:"Clear Errors.vi"("error in (no error)"=w103) -> ()  [unwired: 6 in, 1 out]
          n84 = Open/Create/Replace File(file path (use dialog)=w99) -> (refnum out=w97:refnum<file>, error out=w98:errorcluster)  [unwired: 5 in, 1 out]
          n85 = Read from Binary File(5:w92, 8:w98, 11:w97) -> (0:w95:errorcluster, 2:w91:T23, 3:w96:refnum<file>)  [unwired: 3 in, 1 out]
          n86 = Unbundle(w91) -> ("MAIL SETTINGS"=w90:T7, "Auto Mail Send"=w88:bool, w87:string)
          n87 = local write "TO (string):"(w87) -> ()
          n88 = local write "Auto Mail Send"(w88) -> ()
          n89 = local write "MAIL SETTINGS"(w90) -> ()
          n90 = Close File(refnum=w96, error in=w95) -> (error out=w94:errorcluster)  [unwired: 1 out]
          n91 = local write "data file error"(w94) -> ()
        }
        frame #5 {
          # "set display status if blank"
          n92 = local read "DISP LAB03-2"() -> (w133:T4)
          n93 = local read "DISP LAB03-1"() -> (w140:T4)
          n94 = local read "DISP LAB02-2"() -> (w147:T4)
          n95 = local read "DISP LAB01-2"() -> (w160:T4)
          n96 = local read "DISP LAB01-1"() -> (w169:T4)
          n97 = local read "DISP LAB02-1"() -> (w154:T4)
          n98 = Unbundle(w133) -> ("STATUS"=w135:string)  [unwired: 2 out]
          n99 = Unbundle(w140) -> ("STATUS"=w142:string)  [unwired: 2 out]
          n100 = Unbundle(w147) -> ("STATUS"=w149:string)  [unwired: 2 out]
          n101 = Unbundle(w154) -> ("STATUS"=w156:string)  [unwired: 2 out]
          n102 = Unbundle(w160) -> ("STATUS"=w163:string)  [unwired: 2 out]
          n103 = Unbundle(w169) -> ("STATUS"=w170:string)  [unwired: 2 out]
          n104 = Equal?(x="", y=w135) -> (x = y?=w137:bool)
          n105 = Equal?(x="", y=w142) -> (x = y?=w144:bool)
          n106 = Equal?(x="", y=w149) -> (x = y?=w151:bool)
          n107 = Equal?(x="", y=w156) -> (x = y?=w158:bool)
          n108 = Equal?(x="", y=w163) -> (x = y?=w165:bool)
          n109 = Equal?(x="", y=w170) -> (x = y?=w172:bool)
          n110 = Select(t="STOP", s=w137, f=w135) -> (s? t:f=w134:string)
          n111 = Select(t="STOP", s=w144, f=w142) -> (s? t:f=w141:string)
          n112 = Select(t="STOP", s=w151, f=w149) -> (s? t:f=w148:string)
          n113 = Select(t="STOP", s=w158, f=w156) -> (s? t:f=w155:string)
          n114 = Select(t="STOP", s=w165, f=w163) -> (s? t:f=w162:string)
          n115 = Select(t="STOP", s=w172, f=w170) -> (s? t:f=w168:string)
          n116 = Bundle(cluster=w133, "STATUS"=w134) -> (w132:T4)  [unwired: 2 in]
          n117 = Bundle(cluster=w140, "STATUS"=w141) -> (w139:T4)  [unwired: 2 in]
          n118 = Bundle(cluster=w147, "STATUS"=w148) -> (w146:T4)  [unwired: 2 in]
          n119 = Bundle(cluster=w154, "STATUS"=w155) -> (w153:T4)  [unwired: 2 in]
          n120 = Bundle(cluster=w160, "STATUS"=w162) -> (w161:T4)  [unwired: 2 in]
          n121 = Bundle(cluster=w169, "STATUS"=w168) -> (w167:T4)  [unwired: 2 in]
          n122 = local write "DISP LAB01-2"(w161) -> ()
          n123 = local write "DISP LAB01-1"(w167) -> ()
          n124 = local write "DISP LAB02-1"(w153) -> ()
          n125 = local write "DISP LAB03-1"(w139) -> ()
          n126 = local write "DISP LAB02-2"(w146) -> ()
          n127 = local write "DISP LAB03-2"(w132) -> ()
          n128 = local read "DISP LAB05-2"() -> (w105:T4)
          n129 = local read "DISP LAB05-1"() -> (w112:T4)
          n130 = local read "DISP LAB04-2"() -> (w114:T4)
          n131 = local read "DISP LAB04-1"() -> (w116:T4)
          n132 = Unbundle(w105) -> ("STATUS"=w107:string)  [unwired: 2 out]
          n133 = Unbundle(w112) -> ("STATUS"=w118:string)  [unwired: 2 out]
          n134 = Unbundle(w114) -> ("STATUS"=w123:string)  [unwired: 2 out]
          n135 = Unbundle(w116) -> ("STATUS"=w128:string)  [unwired: 2 out]
          n136 = Equal?(x="", y=w107) -> (x = y?=w109:bool)
          n137 = Equal?(x="", y=w118) -> (x = y?=w120:bool)
          n138 = Equal?(x="", y=w123) -> (x = y?=w125:bool)
          n139 = Equal?(x="", y=w128) -> (x = y?=w130:bool)
          n140 = Select(t="STOP", s=w109, f=w107) -> (s? t:f=w106:string)
          n141 = Select(t="STOP", s=w120, f=w118) -> (s? t:f=w117:string)
          n142 = Select(t="STOP", s=w125, f=w123) -> (s? t:f=w122:string)
          n143 = Select(t="STOP", s=w130, f=w128) -> (s? t:f=w127:string)
          n144 = Bundle(cluster=w105, "STATUS"=w106) -> (w104:T4)  [unwired: 2 in]
          n145 = Bundle(cluster=w112, "STATUS"=w117) -> (w111:T4)  [unwired: 2 in]
          n146 = Bundle(cluster=w114, "STATUS"=w122) -> (w113:T4)  [unwired: 2 in]
          n147 = Bundle(cluster=w116, "STATUS"=w127) -> (w115:T4)  [unwired: 2 in]
          n148 = local write "DISP LAB05-2"(w104) -> ()
          n149 = local write "DISP LAB05-1"(w111) -> ()
          n150 = local write "DISP LAB04-1"(w115) -> ()
          n151 = local write "DISP LAB04-2"(w113) -> ()
        }
        frame #6 {
          # "initialise analog input express vi's"
          n152 = for {
            N: 2.0 -> [_]
            n153 = call "sub vi - analog 1st setup v1.vi"() -> ("Error USB #0"=w178:bool, "Error USB #1"=w177:bool, "Error USB #2"=w176:bool)  [unwired: 9 in, 4 out]
            n154 = local write "Error USB #2"(w176) -> ()
            n155 = local write "Error USB #1"(w177) -> ()
            n156 = And(x=w178, y=w177) -> (x .and. y?=w180:bool)
            n157 = local write "Error USB #0"(w178) -> ()
            n158 = And(x=w180, y=w176) -> (x .and. y?=w179:bool)
            n159 = local write "Simulate IND"(w179) -> ()
            n160 = local write "simulate"(w179) -> ()
            n161 = local write "Reset Measuring"(FALSE) -> ()
          }
        }
        frame #7 {
          # "get initial temperature values"
          n162 = stacked-sequence {
            frame #0 {
              w185 = T12 {"T1 Live"=20.0, "T1 Neut"=20.0, "T2 Live"=20.0, "T2 Neut"=20.0, "ID"=6.0, "ER"=10.0} ("LAB01 TEMP")
              n163 = local write "LAB deg C"(w185) -> ()
              n164 = global write "Global display 4.vi" "LAB deg C"(w185) -> ()
              n165 = local write "OFF amps"(1.5) -> ()
              n166 = local write "ON amps"(20.0) -> ()
              n167 = local write "VOLTS"(250.0) -> ()
              n168 = local write "PF"(0.5) -> ()
            }
            frame #1 {
              w224 = TRUE
              n169 = local read "simulate"() -> (w186:bool)
              n170 = local write "Panel #"(0) -> ()
              n171 = case shown="True" w186 {
                frame False {
                }
                frame True {
                  w226 = 20
                  n172 = local write "Ambient Volts"(2.92) -> ()
                  n173 = global write "Global display 3.vi" "Ref deg C"(w226) -> ()
                  n174 = local write "Ref deg C"(w226) -> ()
                }
              }
              n175 = call "sub vi - GET ALL TEMP v6.vi"("LA01-EN"=w224, "simulate"=w186, "LA02-EN"=w224, "LA03-EN"=w224, "LA04-EN"=w224, "LA05-EN"=w224, "Gen Cal Value"=1) -> ("LA01 TEMP"=w222:T24, "LA02 TEMP"=w215:T24, "LA03 TEMP"=w208:T24, "LA04 TEMP"=w201:T24, "LA05 TEMP"=w194:T24)  [unwired: 3 in, 1 out]
              n176 = local write "LAB05 TEMP"(w194) -> ()
              n177 = local write "LAB04 TEMP"(w201) -> ()
              n178 = local write "LAB01 TEMP"(w222) -> ()
              n179 = local write "LAB02 TEMP"(w215) -> ()
              n180 = local write "LAB03 TEMP"(w208) -> ()
              n181 = Unbundle(w208) -> ("T1"=w205:dbl, "T2"=w204:dbl, "T3"=w203:dbl, "T4"=w202:dbl)  [unwired: 2 out]
              n182 = Unbundle(w222) -> ("T1"=w220:dbl, "T2"=w219:dbl, "T3"=w218:dbl, "T4"=w217:dbl)  [unwired: 2 out]
              n183 = Unbundle(w215) -> ("T1"=w212:dbl, "T2"=w211:dbl, "T3"=w210:dbl, "T4"=w209:dbl)  [unwired: 2 out]
              n184 = Unbundle(w201) -> ("T1"=w199:dbl, "T2"=w198:dbl, "T3"=w197:dbl, "T4"=w196:dbl)  [unwired: 2 out]
              n185 = Unbundle(w194) -> ("T1"=w192:dbl, "T2"=w191:dbl, "T3"=w190:dbl, "T4"=w189:dbl)  [unwired: 2 out]
              n186 = local read "TEMP LA05"() -> (w193:T9)
              n187 = local read "TEMP LA04"() -> (w200:T9)
              n188 = local read "TEMP LA02"() -> (w214:T9)
              n189 = local read "TEMP LA03"() -> (w207:T9)
              n190 = local read "TEMP LA01"() -> (w221:T9)
              n191 = Bundle(cluster=w207, "TL-1"=w205, "TN-1"=w204, "TL-2"=w203, "TN-2"=w202) -> (w206:T9)  [unwired: 4 in]
              n192 = Bundle(cluster=w221, "TL-1"=w220, "TN-1"=w219, "TL-2"=w218, "TN-2"=w217) -> (w216:T9)  [unwired: 4 in]
              n193 = Bundle(cluster=w214, "TL-1"=w212, "TN-1"=w211, "TL-2"=w210, "TN-2"=w209) -> (w213:T9)  [unwired: 4 in]
              n194 = Bundle(cluster=w200, "TL-1"=w199, "TN-1"=w198, "TL-2"=w197, "TN-2"=w196) -> (w195:T9)  [unwired: 4 in]
              n195 = Bundle(cluster=w193, "TL-1"=w192, "TN-1"=w191, "TL-2"=w190, "TN-2"=w189) -> (w188:T9)  [unwired: 4 in]
              n196 = local write "TEMP LA03"(w206) -> ()
              n197 = local write "TEMP LA01"(w216) -> ()
              n198 = local write "TEMP LA02"(w213) -> ()
              n199 = local write "TEMP LA05"(w188) -> ()
              n200 = local write "TEMP LA04"(w195) -> ()
            }
            frame #2 {
              w235 = 0
              n201 = local read "LAB01 TEMP"() -> (w237:T12)
              n202 = local read "SIG LAB01-2"() -> (w232:T2)
              n203 = Unbundle By Name(w237) -> ("T1 Live"=w230:dbl, "T1 Neut"=w229:dbl, "T2 Live"=w228:dbl, "T2 Neut"=w227:dbl)  [unwired: 2 out]
              n204 = local read "SIG LAB01-1"() -> (w234:T2)
              n205 = local read "TEMP LA01"() -> (w238:T9)
              n206 = Bundle By Name(cluster=w238, "TL-1"=w230, "TN-1"=w229, "TL-2"=w228, "TN-2"=w227, "TL -1COUNT"=w235, "TN-1 COUNT"=w235, "TL-2 COUNT"=w235, "TN-2 COUNT"=w235) -> (w236:T9)
              n207 = Bundle(cluster=w234, "Tmp Live"=w230, "Tmp Neut"=w229) -> (w233:T2)  [unwired: 3 in]
              n208 = Bundle(cluster=w232, "Tmp Live"=w228, "Tmp Neut"=w227) -> (w231:T2)  [unwired: 3 in]
              n209 = local write "SIG LAB01-2"(w231) -> ()
              n210 = local write "SIG LAB01-1"(w233) -> ()
              n211 = local write "TEMP LA01"(w236) -> ()
            }
            frame #3 {
              w247 = 0
              n212 = local read "LAB02 TEMP"() -> (w249:T12)
              n213 = Unbundle By Name(w249) -> ("T1 Live"=w242:dbl, "T1 Neut"=w241:dbl, "T2 Live"=w240:dbl, "T2 Neut"=w239:dbl)  [unwired: 2 out]
              n214 = local read "SIG LAB02-1"() -> (w246:T2)
              n215 = local read "SIG LAB02-2"() -> (w245:T2)
              n216 = local read "TEMP LA02"() -> (w250:T9)
